vi "solar_type Set Type.vi"(7 "Enum Names":string[](array[string]), 8 "Name":string, 9 "Type":T1) -> (1 "error out":errorcluster, 3 "Variant":variant)   [LabVIEW 2018]
doc: "This VI returns the data type of the variant. Not all data types are supported. Array of clusters are not supported."
uses:
  <vilib>/Utility/Data Type/NI_Data Type.lvlib
  <vilib>/Utility/Data Type/Type Definitions/Memory Type.ctl
  <vilib>/Utility/Data Type/Type Definitions/Memory Info.ctl
  solar_type Item Type.ctl
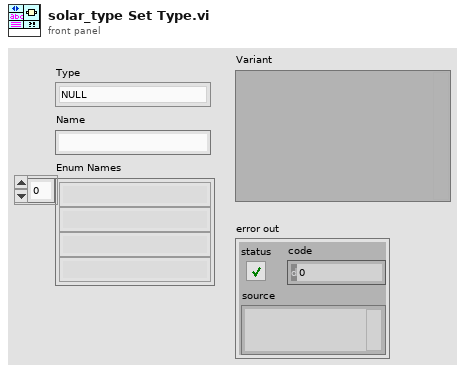
[diagram p1: front panel]
types:
  T1 = typedef "solar_type Item Type.ctl" = enum16{"NULL", "UNKNOWN", "CLUSTER", "I8", "I16", "I32", "I64", "U8", "U16", "U32", "U64", "U8_ENUM", "U16_ENUM", "U32_ENUM", "SGL", "DBL", "BOOLEAN", "STRING", "PATH", "VISA", "TAG", "TIME", "I8_1D", "I16_1D", "I32_1D", "I64_1D", "U8_1D", "U16_1D", "U32_1D", "U64_1D", "U8_ENUM_1D", "U16_ENUM_1D", "U32_ENUM_1D", "SGL_1D", "DBL_1D", "BOOLEAN_1D", "STRING_1D", "PATH_1D", "VISA_1D", "TAG_1D", "TIME_1D", "I8_2D", "I16_2D", "I32_2D", "I64_2D", "U8_2D", "U16_2D", "U32_2D", "U64_2D", "U8_ENUM_2D", "U16_ENUM_2D", "U32_ENUM_2D", "SGL_2D", "DBL_2D", "BOOLEAN_2D", "STRING_2D", "PATH_2D", "VISA_2D", "TAG_2D", "TIME_2D"}
  T2 = typedef "NI_Data Type.lvlib/Memory Info.ctl" = cluster{"Type":T3, "Size":u32}
  T3 = typedef "NI_Data Type.lvlib/Memory Type.ctl" = enum16{"Variable", "Fixed", "Bounded"}
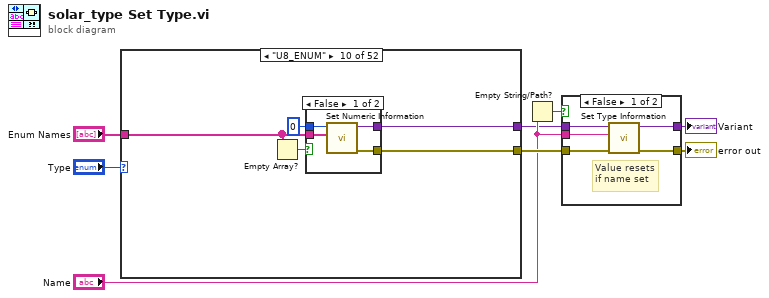
[diagram p0: block diagram]
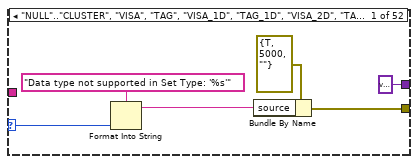
[diagram p3: hidden frame]
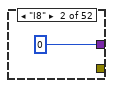
[diagram p4: hidden frame]
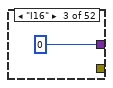
[diagram p5: hidden frame]
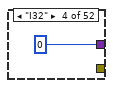
[diagram p6: hidden frame]
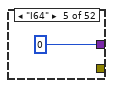
[diagram p7: hidden frame]
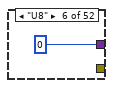
[diagram p8: hidden frame]
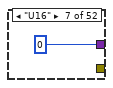
[diagram p9: hidden frame]
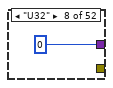
[diagram p10: hidden frame]
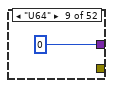
[diagram p11: hidden frame]
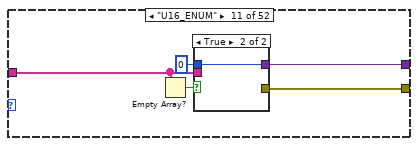
[diagram p13: hidden frame]
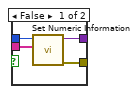
[diagram p14: hidden frame]
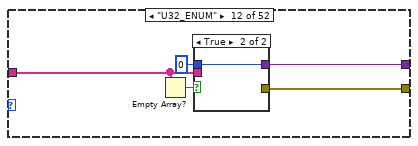
[diagram p15: hidden frame]
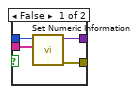
[diagram p16: hidden frame]
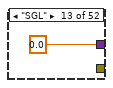
[diagram p17: hidden frame]
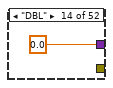
[diagram p18: hidden frame]
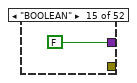
[diagram p19: hidden frame]
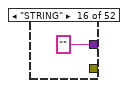
[diagram p20: hidden frame]
diagram:
  n1 = case shown="\"U8_ENUM\"" "Type" {
    selector: "Type" -> [w11 _ _ _ _ _ _ _ _ _ _ _ _ _ _ _ _ _ _ _ _ _ _ _ _ _ _ _ _ _ _ _ _ _ _ _ _ _ _ _ _ _ _ _ _ _ _ _ _ _ _ _]
    tunnel: [w10 _ _ _ _ _ _ _ _ w25 w35 w45 _ _ _ _ _ _ _ _ _ _ _ _ _ _ w69 w83 w97 _ _ _ _ _ _ _ _ _ _ _ _ _ _ w126 w141 w156 _ _ _ _ _ _] -> w6
    tunnel: [variant ("Variant") i8 0 i16 0 0 i64 0 u8 0 u16 0 u32 0 u64 0 w26 w36 w46 sgl 0.0 0.0 FALSE "" path "" timestamp(0 s since 1904-01-01) i8[] [] i16[] [] i32[] [] i64[] [] u8[] [] u16[] [] u32[] [] u64[] [] w68 w82 w96 sgl[] [] dbl[] [] bool[] [] string[] [] path[] [] timestamp[] [] i8[][] [] i16[][] [] i32[][] [] i64[][] [] u8[][] [] u16[][] [] u32[][] [] u64[][] [] w125 w140 w155 sgl[][] [] dbl[][] [] bool[][] [] string[][] [] path[][] [] timestamp[][] []] -> w4
    tunnel: "Enum Names" -> [_ _ _ _ _ _ _ _ _ w24 w34 w44 _ _ _ _ _ _ _ _ _ _ _ _ _ _ w67 w81 w95 _ _ _ _ _ _ _ _ _ _ _ _ _ _ w124 w139 w154 _ _ _ _ _ _]
    frame "NULL".."CLUSTER", "VISA", "TAG", "VISA_1D", "TAG_1D", "VISA_2D", "TAG_2D" {
      n2 = Format Into String(format string="Data type not supported in Set Type: '%s'" ("source"), w11) -> (resulting string=w14:string)  [unwired: 2 in, 1 out]
      n3 = Bundle By Name(cluster=errorcluster {"status"=TRUE, "code"=5000, "source"=""} ("error out"), "source"=w14) -> (w10:errorcluster)
    }
    frame "I8" {
    }
    frame "I16" {
    }
    frame "I32" {
    }
    frame "I64" {
    }
    frame "U8" {
    }
    frame "U16" {
    }
    frame "U32" {
    }
    frame "U64" {
    }
    frame "U8_ENUM" {
      n4 = Empty Array?(array=w24) -> (empty?=w23:bool)
      n5 = case shown="False" w23 {
        tunnel: u8 0 -> [w31 w32]
        tunnel: [w30 w32] -> w26
        tunnel: [w29 _] -> w25
        tunnel: w24 -> [w28 _]
        frame False {
          n6 = call <vilib>:"Set Numeric Information.vi"("Enum Names"=w28, "Variant in"=w31) -> ("error out"=w29:errorcluster, "Variant out"=w30:variant)  [unwired: 8 in]
        }
        frame True {
        }
      }
    }
    frame "U16_ENUM" {
      n7 = Empty Array?(array=w34) -> (empty?=w33:bool)
      n8 = case shown="True" w33 {
        tunnel: u16 0 -> [w41 w42]
        tunnel: [w40 w42] -> w36
        tunnel: [w39 _] -> w35
        tunnel: w34 -> [w38 _]
        frame False {
          n9 = call <vilib>:"Set Numeric Information.vi"("Enum Names"=w38, "Variant in"=w41) -> ("error out"=w39:errorcluster, "Variant out"=w40:variant)  [unwired: 8 in]
        }
        frame True {
        }
      }
    }
    frame "U32_ENUM" {
      n10 = Empty Array?(array=w44) -> (empty?=w43:bool)
      n11 = case shown="True" w43 {
        tunnel: u32 0 -> [w51 w52]
        tunnel: [w50 w52] -> w46
        tunnel: [w49 _] -> w45
        tunnel: w44 -> [w48 _]
        frame False {
          n12 = call <vilib>:"Set Numeric Information.vi"("Enum Names"=w48, "Variant in"=w51) -> ("error out"=w49:errorcluster, "Variant out"=w50:variant)  [unwired: 8 in]
        }
        frame True {
        }
      }
    }
    frame "SGL" {
    }
    frame "DBL" {
    }
    frame "BOOLEAN" {
    }
    frame "STRING" {
    }
    frame "PATH" {
    }
    frame "TIME" {
    }
    frame "I8_1D" {
    }
    frame "I16_1D" {
    }
    frame "I32_1D" {
    }
    frame "I64_1D" {
    }
    frame "U8_1D" {
    }
    frame "U16_1D" {
    }
    frame "U32_1D" {
    }
    frame "U64_1D" {
    }
    frame "U8_ENUM_1D" {
      w72 = u8[] []
      n13 = Index Array(array=w72) -> (element=w71:u8)  [unwired: 1 in]
      n14 = Empty Array?(array=w67) -> (empty?=w75:bool)
      n15 = case shown="True" w75 {
        tunnel: w71 -> [w79 w80]
        tunnel: [w78 w80] -> w74
        tunnel: [w77 _] -> w70
        tunnel: w67 -> [w76 _]
        frame False {
          n16 = call <vilib>:"Set Numeric Information.vi"("Enum Names"=w76, "Variant in"=w79) -> ("error out"=w77:errorcluster, "Variant out"=w78:variant)  [unwired: 8 in]
        }
        frame True {
        }
      }
      n17 = call <vilib>:"Set Array Information.vi"("error in (no error)"=w70, "Array Lengths"=T2[] [{"Type"=enum."Variable", "Size"=0}], "Array Element"=w74, "Variant in"=w72) -> ("error out"=w69:errorcluster, "Variant out"=w68:variant)  [unwired: 6 in]
    }
    frame "U16_ENUM_1D" {
      w86 = u16[] []
      n18 = Index Array(array=w86) -> (element=w85:u16)  [unwired: 1 in]
      n19 = Empty Array?(array=w81) -> (empty?=w89:bool)
      n20 = case shown="True" w89 {
        tunnel: w85 -> [w93 w94]
        tunnel: [w92 w94] -> w88
        tunnel: [w91 _] -> w84
        tunnel: w81 -> [w90 _]
        frame False {
          n21 = call <vilib>:"Set Numeric Information.vi"("Enum Names"=w90, "Variant in"=w93) -> ("error out"=w91:errorcluster, "Variant out"=w92:variant)  [unwired: 8 in]
        }
        frame True {
        }
      }
      n22 = call <vilib>:"Set Array Information.vi"("error in (no error)"=w84, "Array Lengths"=T2[] [{"Type"=enum."Variable", "Size"=0}], "Array Element"=w88, "Variant in"=w86) -> ("error out"=w83:errorcluster, "Variant out"=w82:variant)  [unwired: 6 in]
    }
    frame "U32_ENUM_1D" {
      w100 = u32[] []
      n23 = Index Array(array=w100) -> (element=w99:u32)  [unwired: 1 in]
      n24 = Empty Array?(array=w95) -> (empty?=w103:bool)
      n25 = case shown="True" w103 {
        tunnel: w99 -> [w107 w108]
        tunnel: [w106 w108] -> w102
        tunnel: [w105 _] -> w98
        tunnel: w95 -> [w104 _]
        frame False {
          n26 = call <vilib>:"Set Numeric Information.vi"("Enum Names"=w104, "Variant in"=w107) -> ("error out"=w105:errorcluster, "Variant out"=w106:variant)  [unwired: 8 in]
        }
        frame True {
        }
      }
      n27 = call <vilib>:"Set Array Information.vi"("error in (no error)"=w98, "Array Lengths"=T2[] [{"Type"=enum."Variable", "Size"=0}], "Array Element"=w102, "Variant in"=w100) -> ("error out"=w97:errorcluster, "Variant out"=w96:variant)  [unwired: 6 in]
    }
    frame "SGL_1D" {
    }
    frame "DBL_1D" {
    }
    frame "BOOLEAN_1D" {
    }
    frame "STRING_1D" {
    }
    frame "PATH_1D" {
    }
    frame "TIME_1D" {
    }
    frame "I8_2D" {
    }
    frame "I16_2D" {
    }
    frame "I32_2D" {
    }
    frame "I64_2D" {
    }
    frame "U8_2D" {
    }
    frame "U16_2D" {
    }
    frame "U32_2D" {
    }
    frame "U64_2D" {
    }
    frame "U8_ENUM_2D" {
      w123 = -1 ("index (row)")
      w129 = u8[][] []
      n28 = Index Array(array=w129, index (row)=w123, index (col)=w123) -> (element=w128:u8)
      n29 = Empty Array?(array=w124) -> (empty?=w132:bool)
      n30 = case shown="True" w132 {
        tunnel: w128 -> [w136 w137]
        tunnel: [w135 w137] -> w131
        tunnel: [w134 _] -> w127
        tunnel: w124 -> [w133 _]
        frame False {
          n31 = call <vilib>:"Set Numeric Information.vi"("Enum Names"=w133, "Variant in"=w136) -> ("error out"=w134:errorcluster, "Variant out"=w135:variant)  [unwired: 8 in]
        }
        frame True {
        }
      }
      n32 = call <vilib>:"Set Array Information.vi"("error in (no error)"=w127, "Array Lengths"=T2[] [{"Type"=enum."Variable", "Size"=0}, {"Type"=enum."Variable", "Size"=0}], "Array Element"=w131, "Variant in"=w129) -> ("error out"=w126:errorcluster, "Variant out"=w125:variant)  [unwired: 6 in]
    }
    frame "U16_ENUM_2D" {
      w138 = -1 ("index (row)")
      w144 = u16[][] []
      n33 = Index Array(array=w144, index (row)=w138, index (col)=w138) -> (element=w143:u16)
      n34 = Empty Array?(array=w139) -> (empty?=w147:bool)
      n35 = case shown="True" w147 {
        tunnel: w143 -> [w151 w152]
        tunnel: [w150 w152] -> w146
        tunnel: [w149 _] -> w142
        tunnel: w139 -> [w148 _]
        frame False {
          n36 = call <vilib>:"Set Numeric Information.vi"("Enum Names"=w148, "Variant in"=w151) -> ("error out"=w149:errorcluster, "Variant out"=w150:variant)  [unwired: 8 in]
        }
        frame True {
        }
      }
      n37 = call <vilib>:"Set Array Information.vi"("error in (no error)"=w142, "Array Lengths"=T2[] [{"Type"=enum."Variable", "Size"=0}, {"Type"=enum."Variable", "Size"=0}], "Array Element"=w146, "Variant in"=w144) -> ("error out"=w141:errorcluster, "Variant out"=w140:variant)  [unwired: 6 in]
    }
    frame "U32_ENUM_2D" {
      w153 = -1 ("index (row)")
      w159 = u32[][] []
      n38 = Index Array(array=w159, index (row)=w153, index (col)=w153) -> (element=w158:u32)
      n39 = Empty Array?(array=w154) -> (empty?=w162:bool)
      n40 = case shown="True" w162 {
        tunnel: w158 -> [w166 w167]
        tunnel: [w165 w167] -> w161
        tunnel: [w164 _] -> w157
        tunnel: w154 -> [w163 _]
        frame False {
          n41 = call <vilib>:"Set Numeric Information.vi"("Enum Names"=w163, "Variant in"=w166) -> ("error out"=w164:errorcluster, "Variant out"=w165:variant)  [unwired: 8 in]
        }
        frame True {
        }
      }
      n42 = call <vilib>:"Set Array Information.vi"("error in (no error)"=w157, "Array Lengths"=T2[] [{"Type"=enum."Variable", "Size"=0}, {"Type"=enum."Variable", "Size"=0}], "Array Element"=w161, "Variant in"=w159) -> ("error out"=w156:errorcluster, "Variant out"=w155:variant)  [unwired: 6 in]
    }
    frame "SGL_2D" {
    }
    frame "DBL_2D" {
    }
    frame "BOOLEAN_2D" {
    }
    frame "STRING_2D" {
    }
    frame "PATH_2D" {
    }
    frame "TIME_2D" {
    }
  }
  n43 = Empty String/Path?(string/path="Name") -> (empty?=w2:bool)
  n44 = case shown="False" w2 {
    tunnel: [w175 w179] -> w7
    tunnel: w6 -> [w176 w179]
    tunnel: "Name" -> [w177 _]
    tunnel: w4 -> [w178 w180]
    tunnel: [w174 w180] -> w3
    frame False {
      # "Value resets\nif name set"
      n45 = call <vilib>:"Set Type Information.vi"("error in (no error)"=w176, "Name"=w177, "Variant in"=w178) -> ("error out"=w175:errorcluster, "Variant out"=w174:variant)  [unwired: 7 in]
    }
    frame True {
    }
  }
  "Variant" <- w3
  "error out" <- w7
